vi "Move Button.vi"(4 "Panel Height":i32, 6 "Panel Width":i32, 7 "Button":refnum<vi>, 8 "error in":errorcluster) -> (0 "error out":errorcluster, 1 "Button Padding":i32)   [LabVIEW 2021, in "Pop-Up.lvlib" / "Popup.lvclass"]
doc: "move the button on the screen to the correct location based on the FP size\n\n<b>Code Developed By:</b> +\nDaniel Coons +\nhttps://github.com/danielcoons/tsc-pop-up"
uses:
  Popup.lvclass
  <vilib>/Utility/miscctls.llb/LVBoundsTypeDef.ctl
  <vilib>/Utility/miscctls.llb/LVPositionTypeDef.ctl
  Popup.lvclass/Popup.ctl
panel:
  out "Bounds":T1
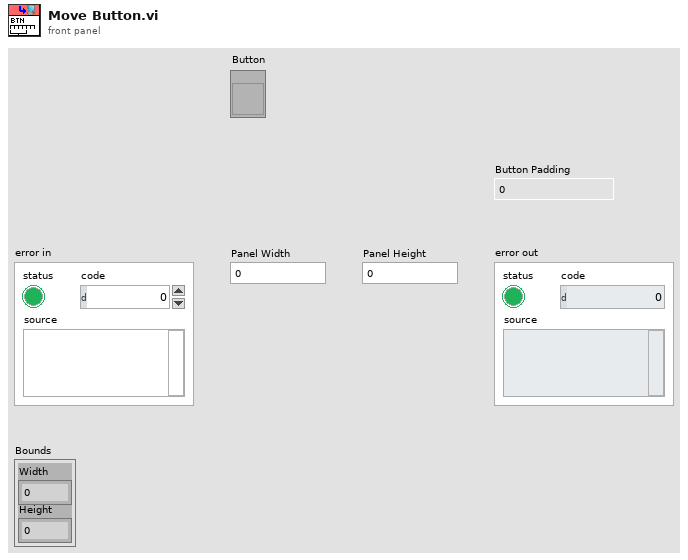
[diagram p1: front panel]
types:
  T1 = typedef "LVBoundsTypeDef.ctl" = cluster{"Width":u32, "Height":u32}
  T2 = typedef "LVPositionTypeDef.ctl" = cluster{"Left":i32, "Top":i32}
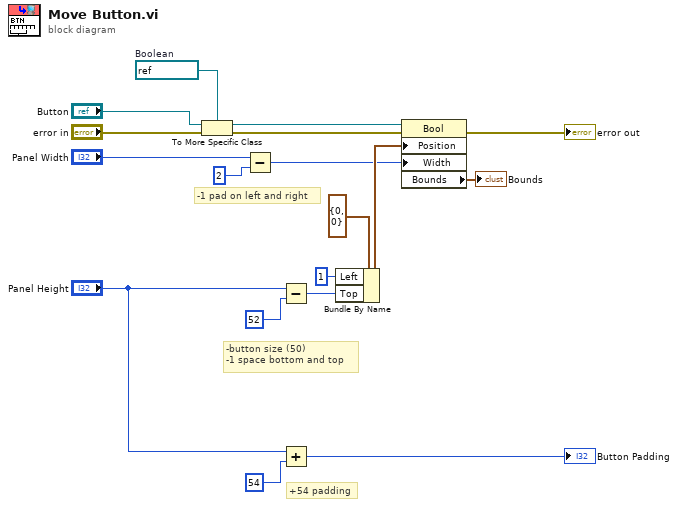
[diagram p0: block diagram]
diagram:
  w5 = refnum<vi> refnum  # Boolean
  # "-button size (50)\n-1 space bottom and top"
  # "-1 pad on left and right"
  # "+54 padding"
  n1 = To More Specific Class(target class=w5, reference="Button", error in="error in") -> (specific class reference=w6:refnum<vi>, error out=w16:errorcluster)
  n2 = Subtract(x="Panel Width", y=2) -> (x-y=w3:i32)
  n3 = Subtract(x="Panel Height", y=52) -> (x-y=w8:i32)
  n4 = Add(x="Panel Height", y=54) -> (x+y=→"Button Padding":i32)
  n5 = Bundle By Name(cluster=T2 {"Left"=0, "Top"=0} ("Position"), "Left"=1, "Top"=w8) -> (w9:T2)
  n6 = property class="Bool"(reference=w6, error in=w16, "Position"=w9, "Width"=w3) -> (error out=→"error out":errorcluster, "Bounds"=→"Bounds":T1)  [unwired: 1 out]
